vi "WriteData.vi"(8 "error in (no error)":errorcluster, 10 "Data":string, 11 "Connection in":refnum<class "Connection.lvclass">) -> (0 "error out":errorcluster, 3 "Connection out":refnum<class "Connection.lvclass">)   [LabVIEW 2022 SP3, in "Connection.lvlib" / "Connection.lvclass"]
uses:
  Connection.lvclass
  C:/Users/jakub/repos/gh/sw4sys/lv-tcp-server-sample/LoggingActor/Source/LoggingActor/LoggingActor/LoggingActor.lvclass
  Connection.lvclass/Connection.ctl
  LoggingActor/Source/LoggingActor/LoggingActor/LoggingActor.lvclass/LoggingActor.ctl
  LoggingActor/Source/LoggingActor/LoggingActor/Read Logger.vi
  Logger/Source/Logger/Logger.lvclass
  TcpSocket/Source/TcpSocket/Connection/Connection.lvclass
  StringUtils/Source/StringUtils/StringUtils.lvlib
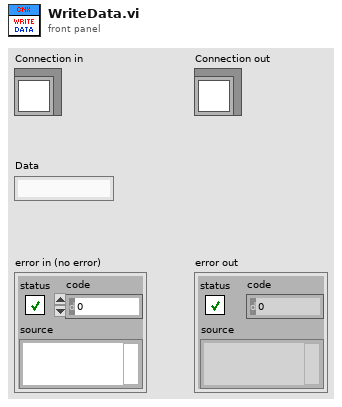
[diagram p1: front panel]
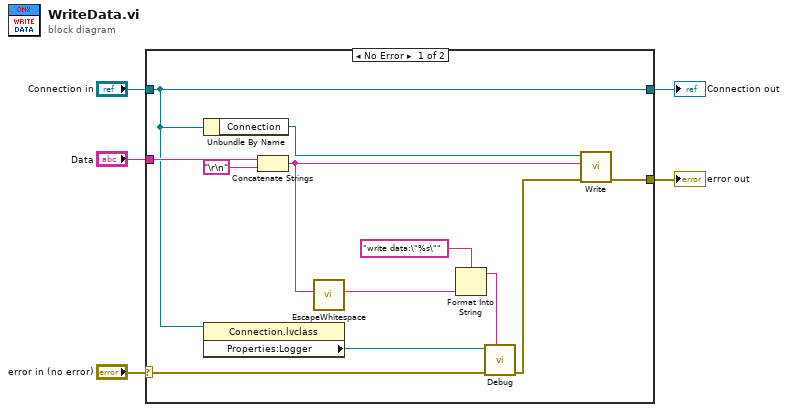
[diagram p0: block diagram]
diagram:
  n1 = case shown="No Error" "error in (no error)" {
    selector: "error in (no error)" -> [w11 w19]
    tunnel: [w17 w19] -> w4
    tunnel: [w13 w18] -> w2
    tunnel: "Connection in" -> [w13 w18]
    tunnel: "Data" -> [w15 _]
    frame No Error {
      n2 = Unbundle By Name(w13) -> ("Connection"=w14:refnum<class "Connection.lvclass">)
      n3 = property class="Connection.lvclass"(reference=w13) -> ("Properties:Logger"=w12:refnum<class "Logger.lvclass">)  [unwired: 1 in, 2 out]
      n4 = Concatenate Strings(w15, "\r\n") -> (w8:string)
      n5 = call "EscapeWhitespace.vi"("InputString"=w8) -> ("EscapedWhitespace"=w6:string)  [unwired: 10 in]
      n6 = Format Into String(format string="write data:\"%s\"", w6) -> (resulting string=w7:string)  [unwired: 2 in, 1 out]
      n7 = call-dynamic "Debug.vi"("Message"=w7, "error in (no error)"=w11, "Logger in"=w12) -> ("error out"=w10:errorcluster)  [unwired: 5 in, 1 out]
      n8 = call-dynamic "Write.vi"("error in (no error)"=w10, "Data"=w8, "Connection in"=w14) -> ("error out"=w17:errorcluster)  [unwired: 7 in, 1 out]
    }
    frame Error {
    }
  }
  "error out" <- w4
  "Connection out" <- w2
